vi "Framework_Initialize.vi"(8 "error in (no error)":errorcluster, 11 "AB_Build in":refnum<class "AB_Build.lvclass">) -> (0 "error out":errorcluster, 1 "helpTopics":string[](array[string]), 2 "pageTitles":string[](array[string]), 3 "AB_Build out":refnum<class "AB_Build.lvclass">, 4 "helpFile":string, 5 "pages":path[](array[path]))   [LabVIEW 2020, in "AB_Build.lvclass"]
uses:
  <vilib>/AppBuilder/AB_Classes/Build/AB_Build.lvclass
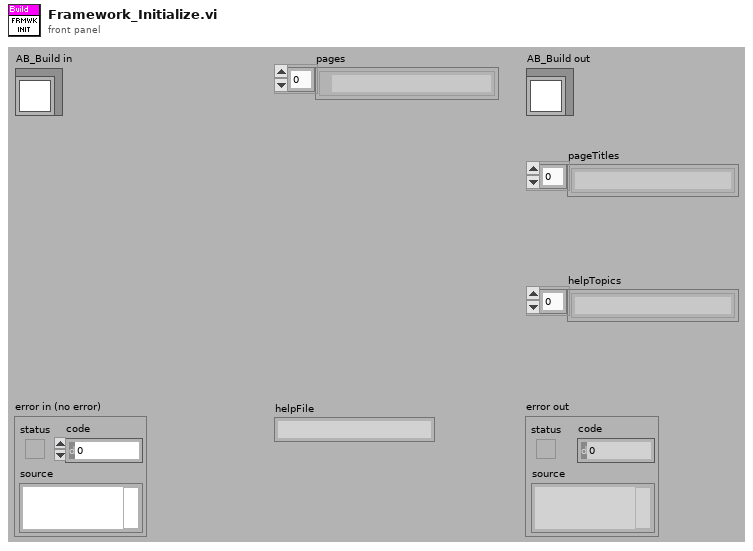
[diagram p1: front panel]
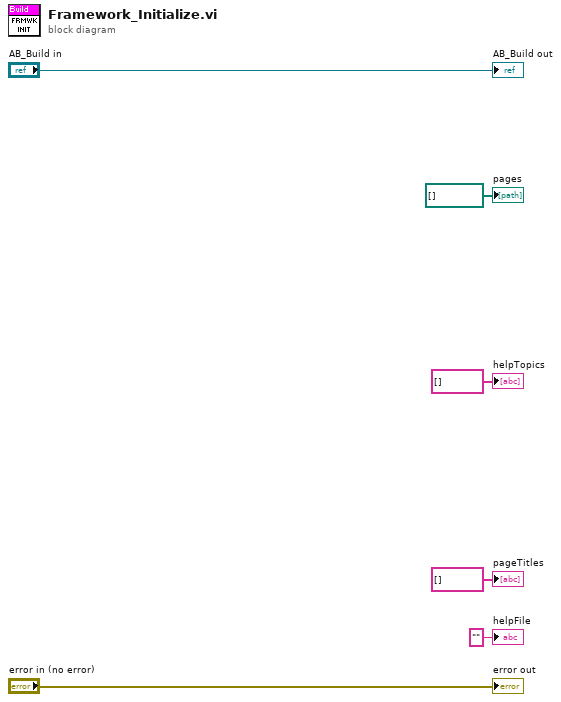
[diagram p0: block diagram]
diagram:
  "error out" <- "error in (no error)"
  "AB_Build out" <- "AB_Build in"
  "pages" <- path[] [] ("pages")
  "helpTopics" <- string[] [] ("helpTopics")
  "pageTitles" <- string[] [] ("pageTitles")
  "helpFile" <- "" ("helpFile")
